vi "Configure Delta Mode.vi"(8 "Voltmeter Integration (NPLC)":dbl=5.0, 9 "Voltage Buffer Size":i32=10, 10 "Voltage Source VISA ID":refnum<visa-resource-name>="GPIB0::7::INSTR", 11 "Current Source Name":string="6221_GPIB12") -> (0 "Error Out Voltmeter":errorcluster, 1 "Error Out Current Source":errorcluster, 2 "Voltmeter Reference Out":refnum<visa-resource-name>="GPIB0::7::INSTR")   [LabVIEW 2020]
uses:
  <instrlib>/Keithley 2182/Keithley 2182.lvlib
panel:
  in  "Error in Current Source":errorcluster
  out "Current Source Reference Out":string="6221_GPIB12"
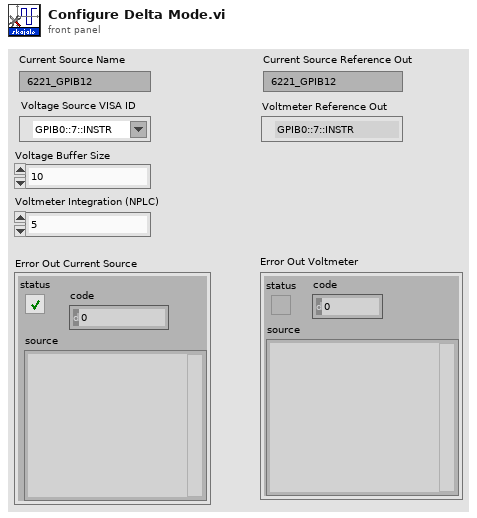
[diagram p1: front panel]
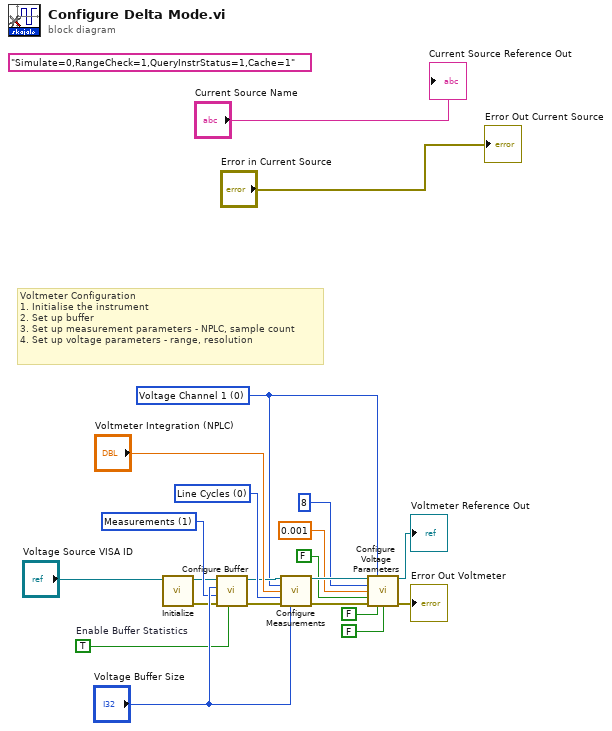
[diagram p0: block diagram]
diagram:
  w4 = 0 items=["Voltage Channel 1", "Voltage Channel 2", "Temperature Channel 1", "Temperature Channel 2"] ("Measurement (0: Voltage Channel 1)")
  w19 = 0 items=["Line Cycles", "Seconds"] ("Integration Rate Units (0: Line Cycles)")
  w15 = 1 items=["None", "Measurements", "Math Calculation"] ("Buffer Source (0: None)")
  w12 = TRUE  # Enable Buffer Statistics
  (unwired) "Simulate=0,RangeCheck=1,QueryInstrStatus=1,Cache=1" ("option string")
  # "Voltmeter Configuration\n1. Initialise the instrument\n2. Set up buffer\n3. Set up measurement parameters - NPLC, sample count\n4. Set up voltage parameters - range, resolution"
  n1 = call <instrlib>:"Initialize.vi"("VISA resource name"="Voltage Source VISA ID") -> ("error out"=w14:errorcluster, "VISA resource name out"=w13:refnum<visa-resource-name>)  [unwired: 9 in]
  n2 = call <instrlib>:"Configure Buffer.vi"("Enable Buffer Statistics (0: Disable)"=w12, "error in (no error)"=w14, "Buffer Source (0: None)"=w15, "Buffer Size (2)"="Voltage Buffer Size", "VISA resource name"=w13) -> ("error out"=w18:errorcluster, "VISA resource name out"=w17:refnum<visa-resource-name>)  [unwired: 5 in]
  n3 = call <instrlib>:"Configure Measurements.vi"("VISA resource name"=w17, "Measurement (0: Voltage Channel 1)"=w4, "Integration Rate (5)"="Voltmeter Integration (NPLC)", "Integration Rate Units (0: Line Cycles)"=w19, "error in (no error)"=w18, "Sample Count (1)"="Voltage Buffer Size") -> ("VISA resource name out"=w11:refnum<visa-resource-name>, "error out"=w10:errorcluster)  [unwired: 8 in]
  n4 = call <instrlib>:"Configure Voltage Parameters.vi"("VISA resource name"=w11, "Measurement (1: Voltage Channel 1)"=w4, "Voltage Resolution (8)"=8, "Range Value (12)"=0.001, "Autorange (T: Enable)"=FALSE, "error in (no error)"=w10, "Enable Ratio (F: Disable)"=FALSE, "Enable Delta (F: Disable)"=FALSE) -> ("VISA resource name out"=→"Voltmeter Reference Out":refnum<visa-resource-name>, "error out"=→"Error Out Voltmeter":errorcluster)  [unwired: 6 in]
  "Error Out Current Source" <- "Error in Current Source"
  "Current Source Reference Out" <- "Current Source Name"
